vi "Find Start XY (SubVI).vi"(0 "Data In":u8, 5 "xStart In":u16, 7 "yStart In":u16, 9 "Fnd?":bool) -> (4 "xStart":u16, 15 "yStart":u16)   [LabVIEW 2015]
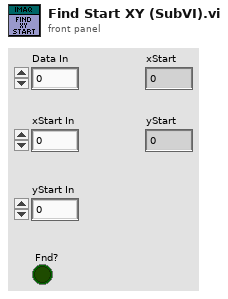
[diagram p1: front panel]
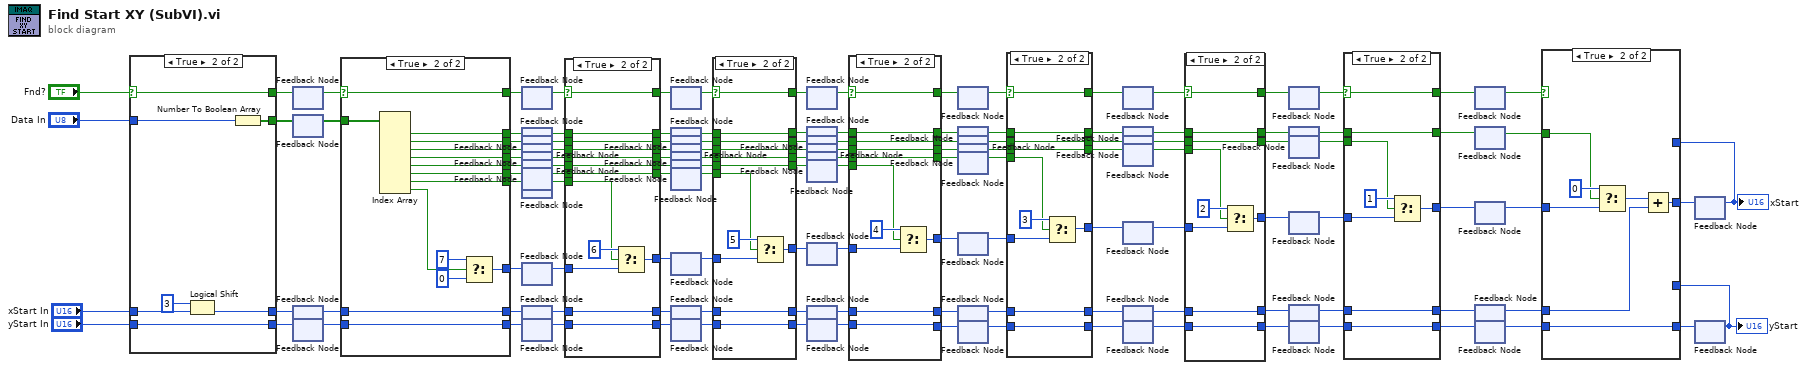
[diagram p0: block diagram]
diagram:
  n1 = case shown="True" "Fnd?" {
    selector: "Fnd?" -> [_ w131]
    tunnel: "Data In" -> [_ w135]
    tunnel: [_ w134] -> w127
    tunnel: "xStart In" -> [_ w133]
    tunnel: "yStart In" -> [_ w132]
    tunnel: [_ w130] -> w106
    tunnel: [_ w132] -> w98
    tunnel: [_ w131] -> w115
    frame False {
    }
    frame True {
      n2 = Logical Shift(y=i16 3, x=w133) -> (x << y=w130:u16)
      n3 = Number To Boolean Array(number=w135) -> (Boolean array=w134:bool[])
    }
  }
  n4 = feedback-in #1(w115) -> ()
  n5 = feedback #1() -> (w60:bool)  [unwired: 1 in]
  n6 = feedback-in #2(w127) -> ()
  n7 = feedback #2() -> (w59:bool[])  [unwired: 1 in]
  n8 = feedback-in #3(w106) -> ()
  n9 = feedback #3() -> (w61:u16)  [unwired: 1 in]
  n10 = feedback-in #4(w98) -> ()
  n11 = feedback #4() -> (w62:u16)  [unwired: 1 in]
  n12 = case shown="True" w60 {
    selector: w60 -> [_ w138]
    tunnel: w59 -> [_ w150]
    tunnel: [_ w147] -> w126
    tunnel: [_ w145] -> w119
    tunnel: [_ w144] -> w64
    tunnel: [_ w143] -> w67
    tunnel: [_ w142] -> w71
    tunnel: [_ w141] -> w76
    tunnel: [_ w140] -> w82
    tunnel: [_ w139] -> w89
    tunnel: [_ w138] -> w114
    tunnel: w61 -> [_ w137]
    tunnel: [_ w137] -> w105
    tunnel: w62 -> [_ w136]
    tunnel: [_ w136] -> w97
    frame False {
    }
    frame True {
      n13 = Index Array(array=w150) -> (element #1=w139:bool, element #2=w140:bool, element #3=w141:bool, element #4=w142:bool, element #5=w143:bool, element #6=w144:bool, element #7=w145:bool, element #8=w146:bool)  [unwired: 8 in]
      n14 = Select(t=u16 7, s=w146, f=u16 0) -> (s? t:f=w147:u16)
    }
  }
  n15 = feedback-in #5(w114) -> ()
  n16 = feedback #5() -> (w50:bool)  [unwired: 1 in]
  n17 = feedback-in #6(w89) -> ()
  n18 = feedback #6() -> (w53:bool)  [unwired: 1 in]
  n19 = feedback-in #7(w82) -> ()
  n20 = feedback #7() -> (w54:bool)  [unwired: 1 in]
  n21 = feedback-in #8(w76) -> ()
  n22 = feedback #8() -> (w55:bool)  [unwired: 1 in]
  n23 = feedback-in #9(w71) -> ()
  n24 = feedback #9() -> (w56:bool)  [unwired: 1 in]
  n25 = feedback-in #10(w67) -> ()
  n26 = feedback #10() -> (w57:bool)  [unwired: 1 in]
  n27 = feedback-in #11(w64) -> ()
  n28 = feedback #11() -> (w58:bool)  [unwired: 1 in]
  n29 = feedback-in #12(w119) -> ()
  n30 = feedback #12() -> (w49:bool)  [unwired: 1 in]
  n31 = feedback-in #13(w126) -> ()
  n32 = feedback #13() -> (w48:u16)  [unwired: 1 in]
  n33 = feedback-in #14(w105) -> ()
  n34 = feedback #14() -> (w51:u16)  [unwired: 1 in]
  n35 = feedback-in #15(w97) -> ()
  n36 = feedback #15() -> (w52:u16)  [unwired: 1 in]
  n37 = case shown="True" w50 {
    selector: w50 -> [_ w159]
    tunnel: w48 -> [_ w162]
    tunnel: [_ w161] -> w125
    tunnel: w49 -> [_ w160]
    tunnel: [_ w159] -> w113
    tunnel: w51 -> [_ w158]
    tunnel: [_ w158] -> w104
    tunnel: w52 -> [_ w157]
    tunnel: [_ w157] -> w96
    tunnel: w53 -> [_ w156]
    tunnel: [_ w156] -> w88
    tunnel: w54 -> [_ w155]
    tunnel: [_ w155] -> w81
    tunnel: w55 -> [_ w154]
    tunnel: [_ w154] -> w75
    tunnel: w56 -> [_ w153]
    tunnel: [_ w153] -> w70
    tunnel: w57 -> [_ w152]
    tunnel: [_ w152] -> w66
    tunnel: w58 -> [_ w151]
    tunnel: [_ w151] -> w63
    frame False {
    }
    frame True {
      n38 = Select(t=u16 6, s=w160, f=w162) -> (s? t:f=w161:u16)
    }
  }
  n39 = feedback-in #16(w113) -> ()
  n40 = feedback #16() -> (w39:bool)  [unwired: 1 in]
  n41 = feedback-in #17(w88) -> ()
  n42 = feedback #17() -> (w42:bool)  [unwired: 1 in]
  n43 = feedback-in #18(w81) -> ()
  n44 = feedback #18() -> (w43:bool)  [unwired: 1 in]
  n45 = feedback-in #19(w75) -> ()
  n46 = feedback #19() -> (w44:bool)  [unwired: 1 in]
  n47 = feedback-in #20(w70) -> ()
  n48 = feedback #20() -> (w45:bool)  [unwired: 1 in]
  n49 = feedback-in #21(w66) -> ()
  n50 = feedback #21() -> (w46:bool)  [unwired: 1 in]
  n51 = feedback-in #22(w63) -> ()
  n52 = feedback #22() -> (w47:bool)  [unwired: 1 in]
  n53 = feedback-in #23(w125) -> ()
  n54 = feedback #23() -> (w38:u16)  [unwired: 1 in]
  n55 = feedback-in #24(w104) -> ()
  n56 = feedback #24() -> (w40:u16)  [unwired: 1 in]
  n57 = feedback-in #25(w96) -> ()
  n58 = feedback #25() -> (w41:u16)  [unwired: 1 in]
  n59 = case shown="True" w39 {
    selector: w39 -> [_ w171]
    tunnel: w38 -> [_ w174]
    tunnel: [_ w173] -> w124
    tunnel: w47 -> [_ w172]
    tunnel: [_ w171] -> w112
    tunnel: w40 -> [_ w170]
    tunnel: [_ w170] -> w103
    tunnel: w41 -> [_ w169]
    tunnel: [_ w169] -> w95
    tunnel: w42 -> [_ w168]
    tunnel: [_ w168] -> w87
    tunnel: w43 -> [_ w167]
    tunnel: [_ w167] -> w80
    tunnel: w44 -> [_ w166]
    tunnel: [_ w166] -> w74
    tunnel: w45 -> [_ w165]
    tunnel: [_ w165] -> w69
    tunnel: w46 -> [_ w164]
    tunnel: [_ w164] -> w65
    frame False {
    }
    frame True {
      n60 = Select(t=u16 5, s=w172, f=w174) -> (s? t:f=w173:u16)
    }
  }
  n61 = feedback-in #26(w112) -> ()
  n62 = feedback #26() -> (w30:bool)  [unwired: 1 in]
  n63 = feedback-in #27(w87) -> ()
  n64 = feedback #27() -> (w33:bool)  [unwired: 1 in]
  n65 = feedback-in #28(w80) -> ()
  n66 = feedback #28() -> (w34:bool)  [unwired: 1 in]
  n67 = feedback-in #29(w74) -> ()
  n68 = feedback #29() -> (w35:bool)  [unwired: 1 in]
  n69 = feedback-in #30(w69) -> ()
  n70 = feedback #30() -> (w36:bool)  [unwired: 1 in]
  n71 = feedback-in #31(w65) -> ()
  n72 = feedback #31() -> (w37:bool)  [unwired: 1 in]
  n73 = feedback-in #32(w124) -> ()
  n74 = feedback #32() -> (w29:u16)  [unwired: 1 in]
  n75 = feedback-in #33(w103) -> ()
  n76 = feedback #33() -> (w31:u16)  [unwired: 1 in]
  n77 = feedback-in #34(w95) -> ()
  n78 = feedback #34() -> (w32:u16)  [unwired: 1 in]
  n79 = case shown="True" w30 {
    selector: w30 -> [_ w182]
    tunnel: w29 -> [_ w185]
    tunnel: [_ w184] -> w123
    tunnel: w37 -> [_ w183]
    tunnel: [_ w182] -> w111
    tunnel: w31 -> [_ w181]
    tunnel: [_ w181] -> w102
    tunnel: w32 -> [_ w180]
    tunnel: [_ w180] -> w94
    tunnel: w33 -> [_ w179]
    tunnel: [_ w179] -> w86
    tunnel: w34 -> [_ w178]
    tunnel: [_ w178] -> w79
    tunnel: w35 -> [_ w177]
    tunnel: [_ w177] -> w73
    tunnel: w36 -> [_ w176]
    tunnel: [_ w176] -> w68
    frame False {
    }
    frame True {
      n80 = Select(t=u16 4, s=w183, f=w185) -> (s? t:f=w184:u16)
    }
  }
  n81 = feedback-in #35(w111) -> ()
  n82 = feedback #35() -> (w22:bool)  [unwired: 1 in]
  n83 = feedback-in #36(w86) -> ()
  n84 = feedback #36() -> (w25:bool)  [unwired: 1 in]
  n85 = feedback-in #37(w79) -> ()
  n86 = feedback #37() -> (w26:bool)  [unwired: 1 in]
  n87 = feedback-in #38(w73) -> ()
  n88 = feedback #38() -> (w27:bool)  [unwired: 1 in]
  n89 = feedback-in #39(w68) -> ()
  n90 = feedback #39() -> (w28:bool)  [unwired: 1 in]
  n91 = feedback-in #40(w123) -> ()
  n92 = feedback #40() -> (w21:u16)  [unwired: 1 in]
  n93 = feedback-in #41(w102) -> ()
  n94 = feedback #41() -> (w23:u16)  [unwired: 1 in]
  n95 = feedback-in #42(w94) -> ()
  n96 = feedback #42() -> (w24:u16)  [unwired: 1 in]
  n97 = case shown="True" w22 {
    selector: w22 -> [_ w192]
    tunnel: w21 -> [_ w195]
    tunnel: [_ w194] -> w120
    tunnel: w28 -> [_ w193]
    tunnel: [_ w192] -> w110
    tunnel: w23 -> [_ w191]
    tunnel: [_ w191] -> w101
    tunnel: w24 -> [_ w190]
    tunnel: [_ w190] -> w93
    tunnel: w25 -> [_ w189]
    tunnel: [_ w189] -> w85
    tunnel: w26 -> [_ w188]
    tunnel: [_ w188] -> w78
    tunnel: w27 -> [_ w187]
    tunnel: [_ w187] -> w72
    frame False {
    }
    frame True {
      n98 = Select(t=u16 3, s=w193, f=w195) -> (s? t:f=w194:u16)
    }
  }
  n99 = feedback-in #43(w110) -> ()
  n100 = feedback #43() -> (w15:bool)  [unwired: 1 in]
  n101 = feedback-in #44(w85) -> ()
  n102 = feedback #44() -> (w18:bool)  [unwired: 1 in]
  n103 = feedback-in #45(w78) -> ()
  n104 = feedback #45() -> (w19:bool)  [unwired: 1 in]
  n105 = feedback-in #46(w72) -> ()
  n106 = feedback #46() -> (w20:bool)  [unwired: 1 in]
  n107 = feedback-in #47(w120) -> ()
  n108 = feedback #47() -> (w14:u16)  [unwired: 1 in]
  n109 = feedback-in #48(w101) -> ()
  n110 = feedback #48() -> (w16:u16)  [unwired: 1 in]
  n111 = feedback-in #49(w93) -> ()
  n112 = feedback #49() -> (w17:u16)  [unwired: 1 in]
  n113 = case shown="True" w15 {
    selector: w15 -> [_ w201]
    tunnel: [_ w205] -> w121
    tunnel: w14 -> [_ w203]
    tunnel: w20 -> [_ w202]
    tunnel: [_ w201] -> w109
    tunnel: w16 -> [_ w200]
    tunnel: [_ w200] -> w100
    tunnel: w17 -> [_ w199]
    tunnel: [_ w199] -> w92
    tunnel: w18 -> [_ w198]
    tunnel: [_ w198] -> w84
    tunnel: w19 -> [_ w197]
    tunnel: [_ w197] -> w77
    frame False {
    }
    frame True {
      n114 = Select(t=u16 2, s=w202, f=w203) -> (s? t:f=w205:u16)
    }
  }
  n115 = feedback-in #50(w109) -> ()
  n116 = feedback #50() -> (w9:bool)  [unwired: 1 in]
  n117 = feedback-in #51(w84) -> ()
  n118 = feedback #51() -> (w12:bool)  [unwired: 1 in]
  n119 = feedback-in #52(w77) -> ()
  n120 = feedback #52() -> (w13:bool)  [unwired: 1 in]
  n121 = feedback-in #53(w121) -> ()
  n122 = feedback #53() -> (w8:u16)  [unwired: 1 in]
  n123 = feedback-in #54(w100) -> ()
  n124 = feedback #54() -> (w10:u16)  [unwired: 1 in]
  n125 = feedback-in #55(w92) -> ()
  n126 = feedback #55() -> (w11:u16)  [unwired: 1 in]
  n127 = case shown="True" w9 {
    selector: w9 -> [_ w209]
    tunnel: [_ w213] -> w122
    tunnel: w8 -> [_ w212]
    tunnel: w13 -> [_ w210]
    tunnel: [_ w209] -> w108
    tunnel: w10 -> [_ w208]
    tunnel: [_ w208] -> w99
    tunnel: w11 -> [_ w207]
    tunnel: [_ w207] -> w91
    tunnel: w12 -> [_ w206]
    tunnel: [_ w206] -> w83
    frame False {
    }
    frame True {
      n128 = Select(t=u16 1, s=w210, f=w212) -> (s? t:f=w213:u16)
    }
  }
  n129 = feedback-in #56(w108) -> ()
  n130 = feedback #56() -> (w4:bool)  [unwired: 1 in]
  n131 = feedback-in #57(w83) -> ()
  n132 = feedback #57() -> (w7:bool)  [unwired: 1 in]
  n133 = feedback-in #58(w122) -> ()
  n134 = feedback #58() -> (w3:u16)  [unwired: 1 in]
  n135 = feedback-in #59(w99) -> ()
  n136 = feedback #59() -> (w5:u16)  [unwired: 1 in]
  n137 = feedback-in #60(w91) -> ()
  n138 = feedback #60() -> (w6:u16)  [unwired: 1 in]
  n139 = feedback #61() -> (w2:u16)  [unwired: 1 in]
  "xStart" <- w2
  n140 = feedback #62() -> (w1:u16)  [unwired: 1 in]
  "yStart" <- w1
  n141 = case shown="True" w4 {
    tunnel: [w215 w222] -> w107
    tunnel: w3 -> [_ w221]
    tunnel: w7 -> [_ w219]
    tunnel: w5 -> [_ w217]
    tunnel: w6 -> [_ w216]
    tunnel: [w214 w216] -> w90
    tunnel: w2 -> [w215 _]
    tunnel: w1 -> [w214 _]
    frame False {
    }
    frame True {
      n142 = Select(t=u16 0, s=w219, f=w221) -> (s? t:f=w218:u16)
      n143 = Add(x=w218, y=w217) -> (x+y=w222:u16)
    }
  }
  n144 = feedback-in #61(w107) -> ()
  n145 = feedback-in #62(w90) -> ()
